vi "deleteme.vi"(8 "error in (no error)":errorcluster) -> (0 "error out":errorcluster)   [LabVIEW 2017]
uses:
  RT/TypeDefs/dataOut.ctl
  RT/TypeDefs/dataIn.ctl
  RT/SubVIs/FGVs/TypeDefs/DataFGVControl.ctl
panel:
  out "XY Graph":cluster{dbl[], dbl[]}[](graph)
  out "DataOut 2":T1
  out "DataIn":T2
  out "DataOut":T1
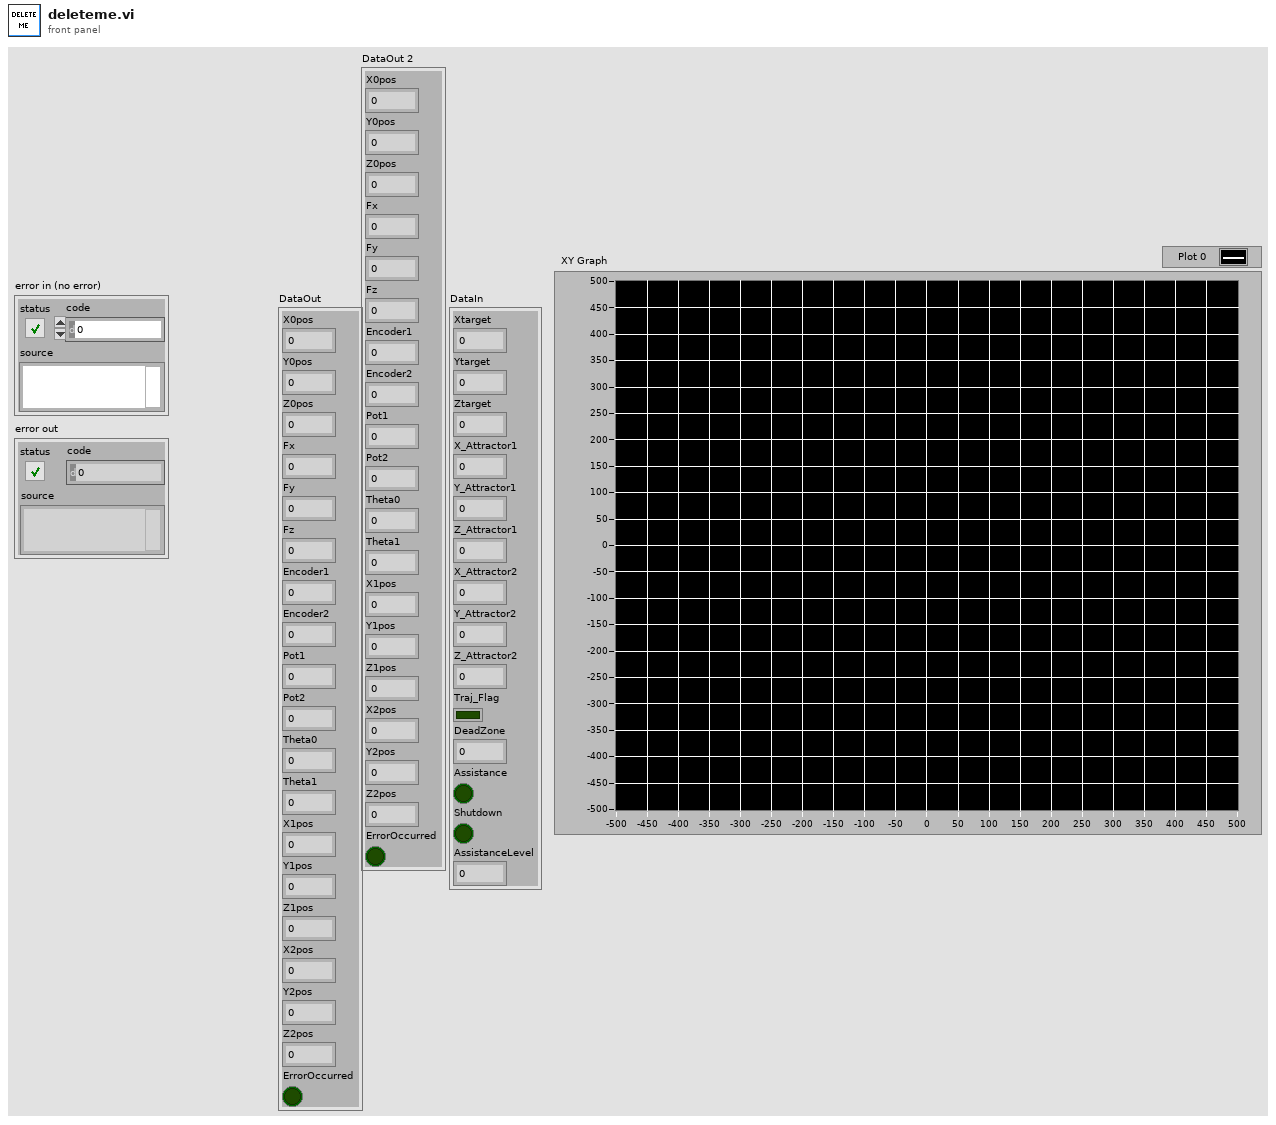
[diagram p1: front panel]
types:
  T1 = typedef "dataOut.ctl" = cluster{"X0pos":dbl, "Y0pos":dbl, "Z0pos":dbl, "Fx":dbl, "Fy":dbl, "Fz":dbl, "Encoder1":i32, "Encoder2":i32, "Pot1":dbl, "Pot2":dbl, "Theta0":dbl, "Theta1":dbl, "X1pos":dbl, "Y1pos":dbl, "Z1pos":dbl, "X2pos":dbl, "Y2pos":dbl, "Z2pos":dbl, "ErrorOccurred":bool}
  T2 = typedef "dataIn.ctl" = cluster{"Xtarget":dbl, "Ytarget":dbl, "Ztarget":dbl, "X_Attractor1":dbl, "Y_Attractor1":dbl, "Z_Attractor1":dbl, "X_Attractor2":dbl, "Y_Attractor2":dbl, "Z_Attractor2":dbl, "Traj_Flag":bool, "DeadZone":dbl, "Assistance":bool, "Shutdown":bool, "AssistanceLevel":dbl}
  T3 = typedef "DataFGVControl.ctl" = enum16{"init", "Set DataOut", "Get DataOut", "Set DataIn", "Get DataIn"}
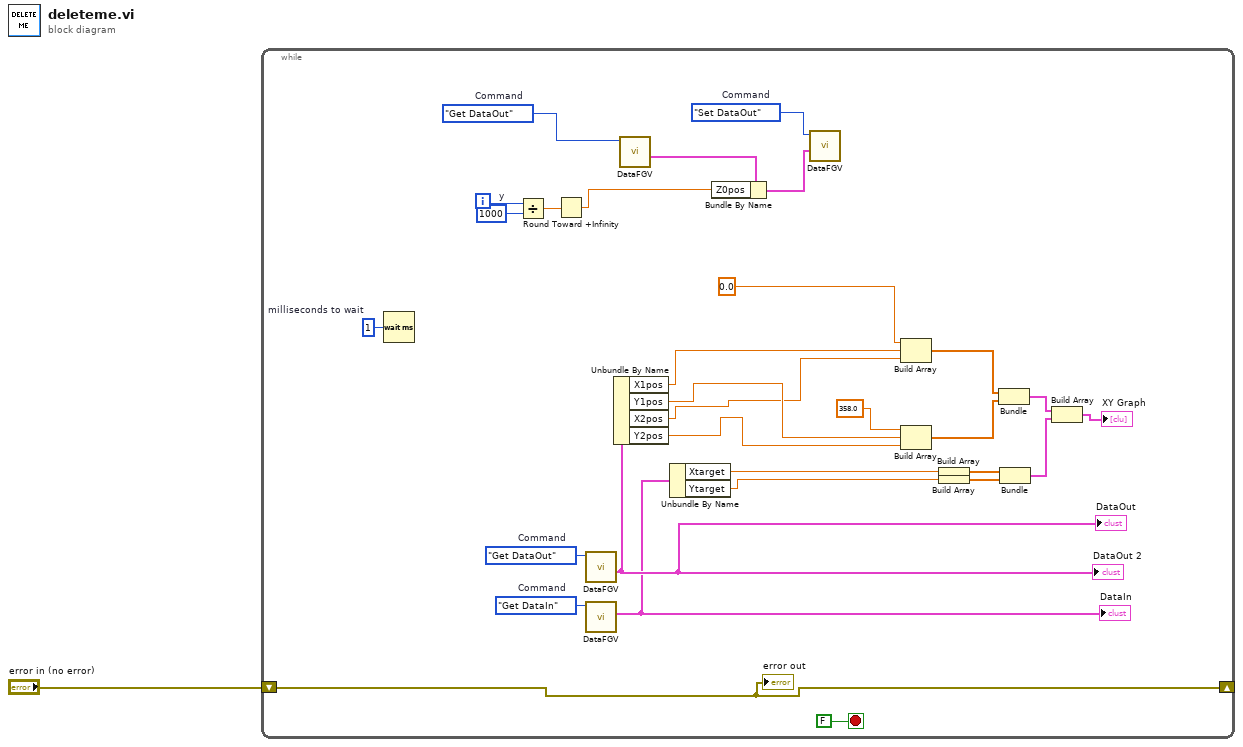
[diagram p0: block diagram]
diagram:
  n1 = while {
    shift-right: [w28] -> _
    shift-left: "error in (no error)" -> [w28]
    i -> [w5]
    stop <- FALSE stop-if-true
    w4 = 1000  # y
    w8 = DataFGVControl."Set DataOut"  # Command
    w9 = DataFGVControl."Get DataOut"  # Command
    w13 = u32 1  # milliseconds to wait
    w30 = DataFGVControl."Get DataIn"  # Command
    w31 = DataFGVControl."Get DataOut"  # Command
    n2 = Wait (ms)(milliseconds to wait=w13) -> ()  [unwired: 1 out]
    n3 = Divide(x=w5, y=w4) -> (x/y=w3:dbl)
    n4 = Round Toward +Infinity(x=w3) -> (ceil(x): smallest int >= x=w2:dbl)
    n5 = call "DataFGV.vi"("Command"=w31) -> ("DataOut"=w18:T1)  [unwired: 8 in, 2 out]
    "DataOut" <- w18
    "DataOut 2" <- w18
    n6 = call "DataFGV.vi"("Command"=w30) -> ("DataIn"=w12:T2)  [unwired: 8 in, 2 out]
    "DataIn" <- w12
    n7 = Unbundle By Name(w18) -> ("X1pos"=w17:dbl, "Y1pos"=w16:dbl, "X2pos"=w15:dbl, "Y2pos"=w14:dbl)
    n8 = call "DataFGV.vi"("Command"=w9) -> ("DataOut"=w7:T1)  [unwired: 8 in, 2 out]
    n9 = Unbundle By Name(w12) -> ("Xtarget"=w11:dbl, "Ytarget"=w10:dbl)
    n10 = Bundle By Name(cluster=w7, "Z0pos"=w2) -> (w6:T1)
    n11 = call "DataFGV.vi"("DataOut"=w6, "Command"=w8) -> ()  [unwired: 7 in, 3 out]
    n12 = Build Array(0.0, w17, w15) -> (w27:dbl[])
    n13 = Build Array(358.0, w16, w14) -> (w26:dbl[])
    n14 = Build Array(w11) -> (w22:dbl[])
    n15 = Build Array(w10) -> (w21:dbl[])
    n16 = Bundle(w27, w26) -> (w23:cluster{dbl[], dbl[]})  [unwired: 1 in]
    n17 = Bundle(w22, w21) -> (w20:cluster{dbl[], dbl[]})  [unwired: 1 in]
    n18 = Build Array(w23, w20) -> (→"XY Graph":cluster{dbl[], dbl[]}[])
    "error out" <- w28
  }
